vi "Enable.vi"(2 "error in (no error)":errorcluster, 3 "Enable Output (T: Enable)":bool=TRUE, 4 "VISA resource name":refnum<visa-resource-name>) -> (0 "error out":errorcluster, 1 "VISA resource name out":refnum<visa-resource-name>)   [LabVIEW 2012]
uses:
  <instrlib>/Keithley 24XX/Keithley 24XX.lvlib
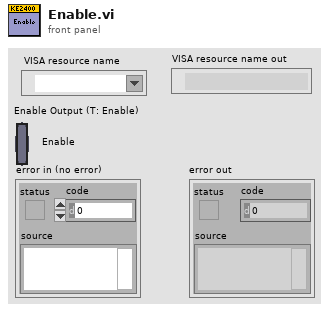
[diagram p1: front panel]
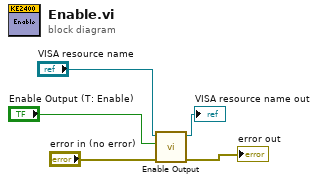
[diagram p0: block diagram]
diagram:
  n1 = call <instrlib>:"Enable Output.vi"("error in (no error)"="error in (no error)", "Enable Output (T: Enable)"="Enable Output (T: Enable)", "VISA resource name"="VISA resource name") -> ("error out"=→"error out":errorcluster, "VISA resource name out"=→"VISA resource name out":refnum<visa-resource-name>)  [unwired: 7 in]
